vi "Plotting Voltage From NI_9219.vi"() -> ()   [LabVIEW 2018]
uses:
  <vilib>/DAQmx/read.llb/DAQmx Read (Analog 1D DBL 1Chan NSamp).vi
  <vilib>/DAQmx/create/channels.llb/DAQmx Create Channel (AI-Voltage-Basic).vi
  <vilib>/DAQmx/configure/timing.llb/DAQmx Timing (Sample Clock).vi
  <vilib>/DAQmx/miscellaneous.llb/DAQmx Fill In Error Info.vi
panel:
  in  "stop":bool
  out "error out":errorcluster
  out "data":dbl[](array[numeric]) format="%0.2f"
  out "Waveform Graph":dbl[](graph)
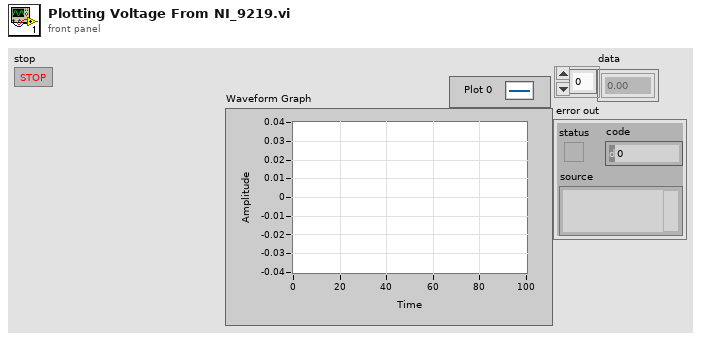
[diagram p1: front panel]
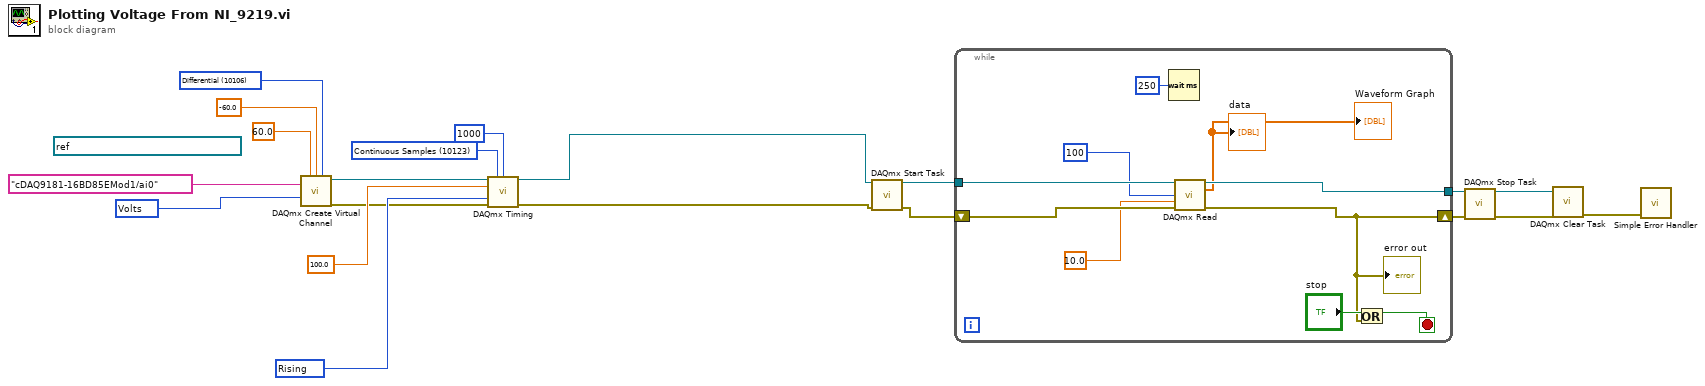
[diagram p0: block diagram]
diagram:
  w12 = 10280 items=["Rising"=10280, "Falling"=10171] ("active edge")
  w15 = 10123 items=["Finite Samples"=10178, "Continuous Samples"=10123, "Hardware Timed Single Point"=12522] ("sample mode")
  w18 = 10106 items=["Default"=-1, "RSE"=10083, "NRSE"=10078, "Differential"=10106, "Pseudodifferential"=12529] ("input terminal configuration")
  w19 = 10348 items=["Volts"=10348, "From Custom Scale"=10065] ("units")
  (unwired) refnum<k21> "MeasureExcitationVoltageTask" ("task in")
  n1 = call-poly <vilib>:"DAQmx Create Virtual Channel.vi"("maximum value"=60.0, "minimum value"=-60.0, "input terminal configuration"=w18, "physical channels"=tag "cDAQ9181-16BD85EMod1/ai0", "units"=w19) -> ("task out"=w4:refnum<k21>, "error out"=w11:errorcluster)  [unwired: 9 in]
  n2 = call-poly <vilib>:"DAQmx Timing.vi"("task/channels in"=w4, "sample mode"=w15, "samples per channel"=1000, "rate"=100.0, "active edge"=w12, "error in"=w11) -> ("task out"=w2:refnum<k21>, "error out"=w1:errorcluster)  [unwired: 8 in]
  n3 = call <vilib>:"DAQmx Start Task.vi"("task/channels in"=w2, "error in"=w1) -> ("task out"=w10:refnum<k21>, "error out"=w3:errorcluster)  [unwired: 12 in]
  n4 = while {
    tunnel: w10 -> [w30]
    tunnel: [w26] -> w9
    shift-right: [w22] -> w8
    shift-left: w3 -> [w29]
    stop <- w23 stop-if-true
    n5 = Wait (ms)(milliseconds to wait=u32 250) -> ()  [unwired: 1 out]
    n6 = call-poly <vilib>:"DAQmx Read.vi"("task/channels in"=w30, "number of samples per channel"=100, "timeout"=10.0, "error in"=w29) -> ("task out"=w26:refnum<k21>, "data"=→"Waveform Graph" →"data":dbl[], "error out"=w22:errorcluster)  [unwired: 9 in]
    "error out" <- w22
    n7 = Or(x="stop", y=w22) -> (x .or. y?=w23:bool)
  }
  n8 = call <vilib>:"DAQmx Stop Task.vi"("task/channels in"=w9, "error in"=w8) -> ("task out"=w7:refnum<k21>, "error out"=w6:errorcluster)  [unwired: 12 in]
  n9 = call <vilib>:"DAQmx Clear Task.vi"("task in"=w7, "error in"=w6) -> ("error out"=w5:errorcluster)  [unwired: 13 in]
  n10 = call <vilib>:"Simple Error Handler.vi"("error in (no error)"=w5) -> ()  [unwired: 4 in, 5 out]
